vi "generateSimulatedData.vi"(8 "error in (no error)":errorcluster, 11 "ILCSim1 in":refnum<class "ILCSim1.lvclass">) -> (0 "error out":errorcluster, 2 "stringRead":string, 3 "ILCSim1 out":refnum<class "ILCSim1.lvclass">)   [LabVIEW 2015, in "ILCSim1.lvclass"]
uses:
  <userlib>/Common/Simulators/ILCSim1/ILCSim1.lvclass
  <userlib>/Common/Simulators/ILCSimulatorSignals/RequestParameters.ctl
  <userlib>/Common/ILC/Configuration/Scan Rates.ctl
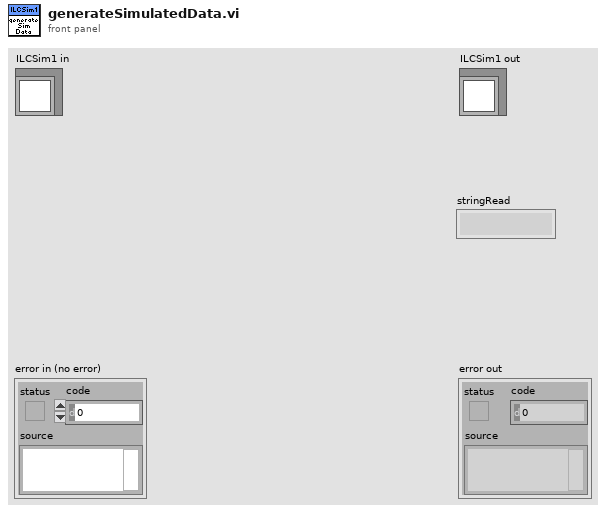
[diagram p1: front panel]
types:
  T1 = typedef "ILCSimulatorSignals.lvlib/RequestParameters.ctl" = cluster{"Time Stamp":timestamp, "answeredIsTrue":bool, "Scan Rate (Hz) ":T2, "Input Channels":enum16{"Channel 0", "3 Channels", "5 Channels"}}
  T2 = typedef "ILCCommon.lvlib/ILCConfiguration.lvlib/Scan Rates.ctl" = enum16{"50", "60", "100", "120", "200", "240", "300", "400", "480", "600", "1200", "2400", "4800"}
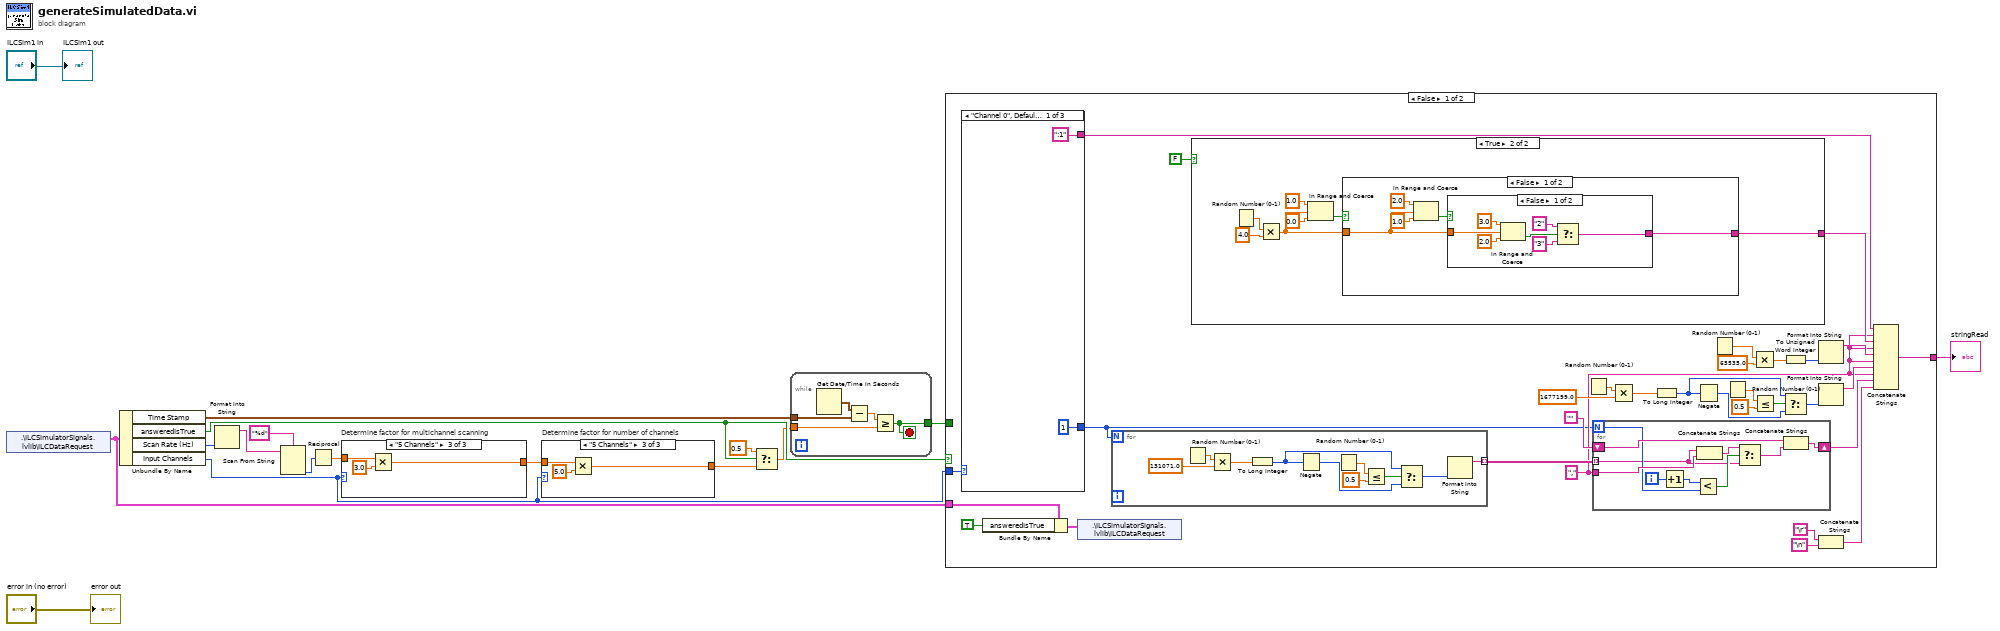
[diagram p0: block diagram]
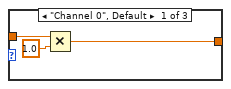
[diagram p2: hidden frame]
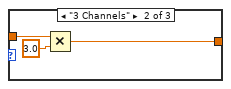
[diagram p3: hidden frame]
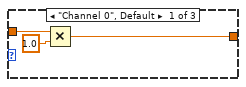
[diagram p4: hidden frame]
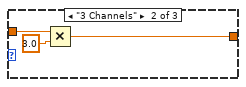
[diagram p5: hidden frame]
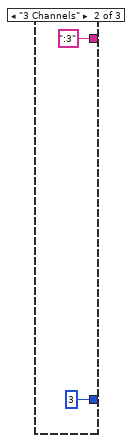
[diagram p6: hidden frame]
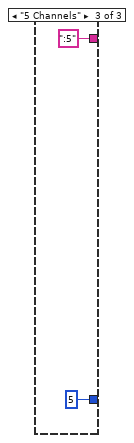
[diagram p7: hidden frame]
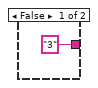
[diagram p8: hidden frame]
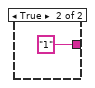
[diagram p9: hidden frame]
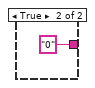
[diagram p10: hidden frame]
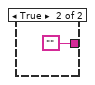
[diagram p11: hidden frame]
diagram:
  n1 = shared-variable ".\\ILCSimulatorSignals.lvlib\\ILCDataRequest"() -> (w14:T1)  [unwired: 1 in, 1 out]
  n2 = Unbundle By Name(w14) -> ("Time Stamp"=w11:timestamp, "answeredIsTrue"=w10:bool, "Scan Rate (Hz)"=w5:T2, "Input Channels"=w1:enum16{"Channel 0", "3 Channels", "5 Channels"})
  n3 = Format Into String(w5) -> (resulting string=w3:string)  [unwired: 3 in, 1 out]
  n4 = Scan From String(format string="%d", input string=w3) -> (output 1=w2:i32)  [unwired: 3 in, 3 out]
  n5 = Reciprocal(x=w2) -> (1/x=w13:dbl)
  n6 = case "Determine factor for multichannel scanning" shown="\"5 Channels\"" w1 {
    tunnel: w13 -> [w19 w23 w25]
    tunnel: [w18 w21 w24] -> w12
    frame "Channel 0", Default {
      n7 = Multiply(x=w19, y=1.0) -> (x*y=w18:dbl)
    }
    frame "3 Channels" {
      n8 = Multiply(x=w23, y=3.0) -> (x*y=w21:dbl)
    }
    frame "5 Channels" {
      n9 = Multiply(x=w25, y=3.0) -> (x*y=w24:dbl)
    }
  }
  n10 = case "Determine factor for number of channels" shown="\"5 Channels\"" w1 {
    tunnel: w12 -> [w28 w32 w34]
    tunnel: [w27 w30 w33] -> w6
    frame "Channel 0", Default {
      n11 = Multiply(x=w28, y=1.0) -> (x*y=w27:dbl)
    }
    frame "3 Channels" {
      n12 = Multiply(x=w32, y=3.0) -> (x*y=w30:dbl)
    }
    frame "5 Channels" {
      n13 = Multiply(x=w34, y=5.0) -> (x*y=w33:dbl)
    }
  }
  n14 = Select(t=0.5, s=w10, f=w6) -> (s? t:f=w9:dbl)
  n15 = while {
    tunnel: w11 -> [w39]
    tunnel: w9 -> [w37]
    tunnel: [w36] -> w8
    stop <- w36 stop-if-true
    n16 = Get Date/Time In Seconds() -> (seconds since 1Jan1904=w40:timestamp)
    n17 = Subtract(x=w40, y=w39) -> (x-y=w38:dbl)
    n18 = Greater Or Equal?(x=w38, y=w37) -> (x >= y?=w36:bool)
  }
  n19 = case shown="False" w10 {
    tunnel: [w51 ""] -> w17
    tunnel: w14 -> [w50 _]
    tunnel: w8 -> [_ _]
    tunnel: w1 -> [w42 _]
    frame False {
      w44 = "," ("string")
      n20 = case shown="\"Channel 0\", Default" w42 {
        tunnel: [":1" ("string") ":3" ("string") ":5" ("string")] -> w47
        tunnel: [1 3 5] -> w41
        frame "Channel 0", Default {
        }
        frame "3 Channels" {
        }
        frame "5 Channels" {
        }
      }
      n21 = Bundle By Name(cluster=w50, "answeredIsTrue"=TRUE) -> (w48:T1)
      n22 = shared-variable ".\\ILCSimulatorSignals.lvlib\\ILCDataRequest"(w48) -> ()  [unwired: 1 in, 1 out]
      n23 = for {
        N: w41 -> [_]
        tunnel: [w110] -> w46 mode=indexing
        n24 = Random Number (0-1)() -> (number: 0 to 1=w111:dbl)
        n25 = Multiply(x=w111, y=131071.0) -> (x*y=w115:dbl)
        n26 = To Long Integer(number=w115) -> (32bit integer=w116:i32)
        n27 = Negate(x=w116) -> (-x=w118:i32)
        n28 = Random Number (0-1)() -> (number: 0 to 1=w113:dbl)
        n29 = Less Or Equal?(x=w113, y=0.5) -> (x <= y?=w117:bool)
        n30 = Select(t=w116, s=w117, f=w118) -> (s? t:f=w119:i32)
        n31 = Format Into String(w119) -> (resulting string=w110:string)  [unwired: 3 in, 1 out]
      }
      n32 = case shown="True" FALSE {
        tunnel: ["3" ("string") w90] -> w71
        frame False {
        }
        frame True {
          n33 = Random Number (0-1)() -> (number: 0 to 1=w95:dbl)
          n34 = Multiply(x=w95, y=4.0) -> (x*y=w89:dbl)
          n35 = In Range and Coerce(upper limit=1.0, x=w89, lower limit=0.0) -> (In Range?=w91:bool)  [unwired: 1 out]
          n36 = case shown="False" w91 {
            tunnel: [w97 "0" ("string")] -> w90
            tunnel: w89 -> [w96 _]
            frame False {
              n37 = In Range and Coerce(upper limit=2.0, x=w96, lower limit=1.0) -> (In Range?=w98:bool)  [unwired: 1 out]
              n38 = case shown="False" w98 {
                tunnel: [w102 "1" ("string")] -> w97
                tunnel: w96 -> [w101 _]
                frame False {
                  n39 = In Range and Coerce(upper limit=3.0, x=w101, lower limit=2.0) -> (In Range?=w105:bool)  [unwired: 1 out]
                  n40 = Select(t="2" ("string"), s=w105, f="3" ("string")) -> (s? t:f=w102:string)
                }
                frame True {
                }
              }
            }
            frame True {
            }
          }
        }
      }
      n41 = Random Number (0-1)() -> (number: 0 to 1=w65:dbl)
      n42 = for {
        N: w41 -> [w76]
        tunnel: w46 -> [w72] mode=indexing
        shift-right: [w81] -> w43
        shift-left: "" -> [w80]
        tunnel: w44 -> [w79]
        i -> [w78]
        n43 = Increment(x=w78) -> (x+1=w77:i32)
        n44 = Less?(x=w77, y=w76) -> (x < y?=w75:bool)
        n45 = Concatenate Strings(w72, w79) -> (w74:string)
        n46 = Select(t=w74, s=w75, f=w72) -> (s? t:f=w73:string)
        n47 = Concatenate Strings(w80, w73) -> (w81:string)
      }
      n48 = Multiply(x=w65, y=1677199.0) -> (x*y=w61:dbl)
      n49 = To Long Integer(number=w61) -> (32bit integer=w60:i32)
      n50 = Negate(x=w60) -> (-x=w58:i32)
      n51 = Random Number (0-1)() -> (number: 0 to 1=w69:dbl)
      n52 = Random Number (0-1)() -> (number: 0 to 1=w63:dbl)
      n53 = Multiply(x=w69, y=65535.0) -> (x*y=w68:dbl)
      n54 = Less Or Equal?(x=w63, y=0.5) -> (x <= y?=w59:bool)
      n55 = To Unsigned Word Integer(number=w68) -> (unsigned 16bit integer=w67:u16)
      n56 = Select(t=w60, s=w59, f=w58) -> (s? t:f=w57:i32)
      n57 = Format Into String(w67) -> (resulting string=w66:string)  [unwired: 3 in, 1 out]
      n58 = Format Into String(w57) -> (resulting string=w56:string)  [unwired: 3 in, 1 out]
      n59 = Concatenate Strings("\r", "\n") -> (w53:string)
      n60 = Concatenate Strings(w47, w44, w71, w44, w66, w44, w56, w44, w43, w53) -> (w51:string)
    }
    frame True {
    }
  }
  "stringRead" <- w17
  "error out" <- "error in (no error)"
  "ILCSim1 out" <- "ILCSim1 in"
